vi "Check Incoming TP Timeouts.vi"(0 "J1939 Cluster":T7, 5 "ref in":T1, 11 "error in":errorcluster) -> (15 "error out":errorcluster)   [LabVIEW 2015, in "J1939 Addon Engine.lvlib"]
uses:
  J1939 Addon Engine.lvlib
  Types/Setup Information Cluster.ctl
  <vilib>/xnet/xnet.llb/XNET Frame CAN.ctl
  <vilib>/xnet/xnet.llb/XNET Frame Type CAN.ctl
  Shared/J1939 Utilities/Types/CAN Outgoing Message Cluster.ctl
  Types/TP List References.ctl
  Types/BAM Buffer Connections List_Ref.ctl
  Types/TP Buffer Connection Cluster.ctl
  Types/Connection Mode Generation Connection Ref.ctl
  Types/Connection Mode Generation Connection Cluster.ctl
  Types/BAM Generation Connections List_Ref.ctl
  Types/BAM Generation Connection Cluster.ctl
  Types/Address Table Reference.ctl
  Types/RQST Lookup Table Reference.ctl
  Types/TP Connections List State.ctl
  SubVIs/TP Buffer Check Timeout on Connections.vi
  SubVIs/Buffer Connections List_Actions.vi
  Shared/J1939 Utilities/SubVIs/TP.Conn Abort.vi
  Shared/J1939 Utilities/Common Conversions.vi
  Shared/J1939 Utilities/SubVIs/Convert J1939 ID to CAN Arb ID.vi
  SubVIs/BAM Buffer Connections List.vi
  Shared/J1939 Utilities/J1939 Utilities.lvlib
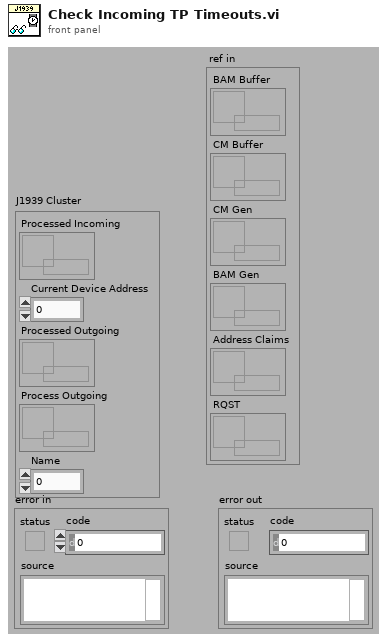
[diagram p1: front panel]
types:
  T1 = typedef "J1939 Addon Engine.lvlib/TP List References.ctl" = cluster{"BAM Buffer":T2, "CM Buffer":T2, "CM Gen":T3, "BAM Gen":T4, "Address Claims":T5, "RQST":T6}
  T2 = typedef "J1939 Addon Engine.lvlib/BAM Buffer Connections List_Ref.ctl" = refnum<data-value>
  T3 = typedef "J1939 Addon Engine.lvlib/Connection Mode Generation Connection Ref.ctl" = refnum<data-value>
  T4 = typedef "J1939 Addon Engine.lvlib/BAM Generation Connections List_Ref.ctl" = refnum<data-value>
  T5 = typedef "J1939 Addon Engine.lvlib/Address Table Reference.ctl" = refnum<data-value>
  T6 = typedef "J1939 Addon Engine.lvlib/RQST Lookup Table Reference.ctl" = refnum<data-value>
  T7 = typedef "J1939 Addon Engine.lvlib/Setup Information Cluster.ctl" = cluster{"Processed Incoming":refnum<queue>, "Current Device Address":u8, "Processed Outgoing":refnum<queue>, "Process Outgoing":refnum<queue>, "Name":u64}
  T8 = typedef "J1939 Addon Engine.lvlib/TP Connections List State.ctl" = enum16{"Add", "Update", "Get", "Remove", "Initialize"}
  T9 = typedef "J1939 Addon Engine.lvlib/TP Buffer Connection Cluster.ctl" = cluster{"Source Address":u8, "Destination Address":u8, "PGN":u32, "Arb ID":u32, "CAN Conversion Index":u32, "Total Expected Bytes":u16, "Total Expected Packets":u8, "Number of Packets Read":u8, "Start Time":u32, "Packets (U8)":u8[], "Timestamp":timestamp}
  T10 = typedef "J1939 Addon Shared.lvlib/J1939 Utilities.lvlib/CAN Outgoing Message Cluster.ctl" = cluster{"Identifier":u32, "Data":u8[]}
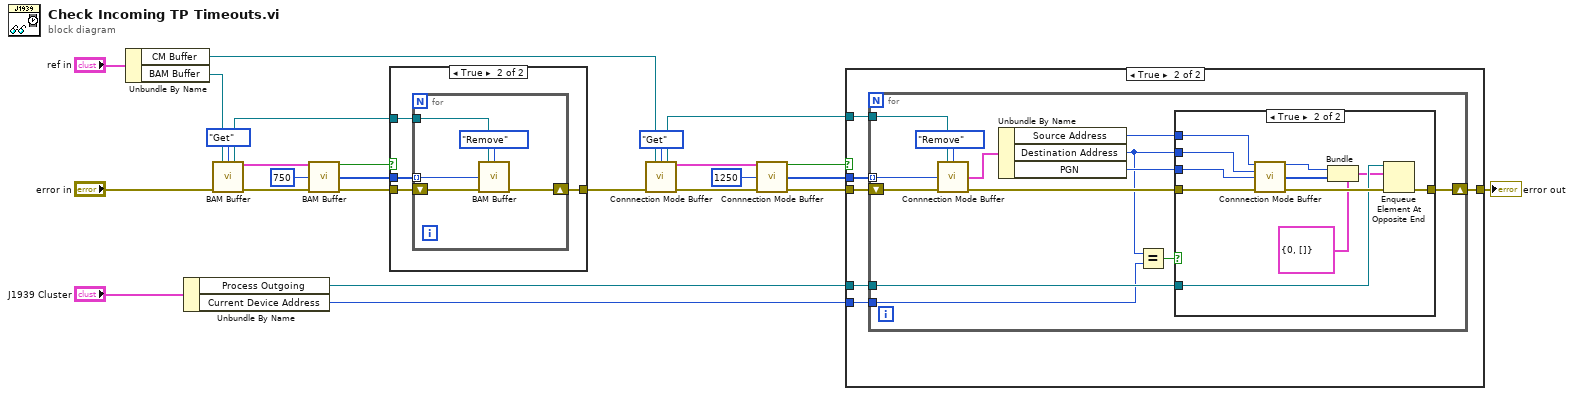
[diagram p0: block diagram]
diagram:
  n1 = Unbundle By Name("ref in") -> ("CM Buffer"=w3:T2, "BAM Buffer"=w4:T2)
  n2 = Unbundle By Name("J1939 Cluster") -> ("Process Outgoing"=w8:refnum<queue>, "Current Device Address"=w1:u8)
  n3 = call-poly "BAM Buffer.vi"("Connections Ref"=w4, "State"=TP_Connections_List_State."Get", "error in (no error)"="error in") -> ("Connections Ref out"=w5:T2, "Connections"=w12:T9[], "error out"=w13:errorcluster)  [unwired: 9 in, 1 out]
  n4 = call-poly "BAM Buffer.vi"("Connections"=w12, "Time Out"=u32 750, "error in (no error)"=w13) -> ("Timed Out Connections?"=w14:bool, "Index Array"=w15:i32[], "error out"=w16:errorcluster)  [unwired: 10 out]
  n5 = case shown="True" w14 {
    tunnel: w15 -> [_ w30]
    tunnel: w16 -> [w26 w29]
    tunnel: [w26 w28] -> w18
    tunnel: w5 -> [_ w27]
    frame False {
    }
    frame True {
      n6 = for {
        tunnel: w30 -> [w34] mode=indexing
        shift-right: [w32] -> w28
        shift-left: w29 -> [w33]
        tunnel: w27 -> [w31]
        n7 = call-poly "BAM Buffer.vi"("Connections Ref"=w31, "State"=TP_Connections_List_State."Remove", "index"=w34, "error in (no error)"=w33) -> ("error out"=w32:errorcluster)  [unwired: 8 in, 3 out]
      }
    }
  }
  n8 = call-poly "Connnection Mode Buffer.vi"("Connections Ref"=w3, "State"=TP_Connections_List_State."Get", "error in (no error)"=w18) -> ("Connections Ref out"=w2:T2, "Connections"=w21:T9[], "error out"=w17:errorcluster)  [unwired: 2 in, 8 out]
  n9 = call-poly "Connnection Mode Buffer.vi"("Connections"=w21, "Time Out"=u32 1250, "error in (no error)"=w17) -> ("Timed Out Connections?"=w24:bool, "Index Array"=w23:i32[], "error out"=w22:errorcluster)  [unwired: 10 out]
  n10 = case shown="True" w24 {
    tunnel: w23 -> [_ w42]
    tunnel: w22 -> [w36 w41]
    tunnel: [w36 w40] -> w25
    tunnel: w8 -> [_ w39]
    tunnel: w2 -> [_ w38]
    tunnel: w1 -> [_ w37]
    frame False {
    }
    frame True {
      n11 = for {
        tunnel: w42 -> [w54] mode=indexing
        shift-right: [w48] -> w40
        shift-left: w41 -> [w55]
        tunnel: w39 -> [w47]
        tunnel: w38 -> [w46]
        tunnel: w37 -> [w45]
        n12 = call-poly "Connnection Mode Buffer.vi"("Connections Ref"=w46, "State"=TP_Connections_List_State."Remove", "index"=w54, "error in (no error)"=w55) -> ("Connection Cluster Out"=w51:T9, "error out"=w52:errorcluster)  [unwired: 1 in, 9 out]
        n13 = Unbundle By Name(w51) -> ("Source Address"=w50:u8, "Destination Address"=w44:u8, "PGN"=w49:u32)
        n14 = Equal?(x=w44, y=w45) -> (x = y?=w43:bool)
        n15 = case shown="True" w43 {
          tunnel: w52 -> [w56 w67]
          tunnel: w50 -> [_ w66]
          tunnel: w44 -> [_ w65]
          tunnel: w49 -> [_ w64]
          tunnel: [w56 w62] -> w48
          tunnel: w47 -> [_ w61]
          frame False {
          }
          frame True {
            n16 = call-poly "Connnection Mode Buffer.vi"("Destination Address"=w66, "Source Address"=w65, "PGN"=w64, "error in (no error)"=w67) -> ("Arb ID"=w60:u32, "Data"=w59:u8[], "error out"=w63:errorcluster)  [unwired: 9 out]
            n17 = Bundle(cluster=T10 {"Identifier"=0, "Data"=[]} ("Data to Send"), "Identifier"=w60, "Data"=w59) -> (w57:T10)
            n18 = Enqueue Element At Opposite End(queue=w61, element=w57, error in (no error)=w63) -> (error out=w62:errorcluster)  [unwired: 3 out]
          }
        }
      }
    }
  }
  "error out" <- w25
